vi "Select Data Items.vi"(10 "Page":i32, 11 "Data":T1(array[cluster])) -> (3 "subarray":string[][](array[string]))   [LabVIEW 2019, in "Full User Interface.lvlib"]
uses:
  Full User Interface.lvlib
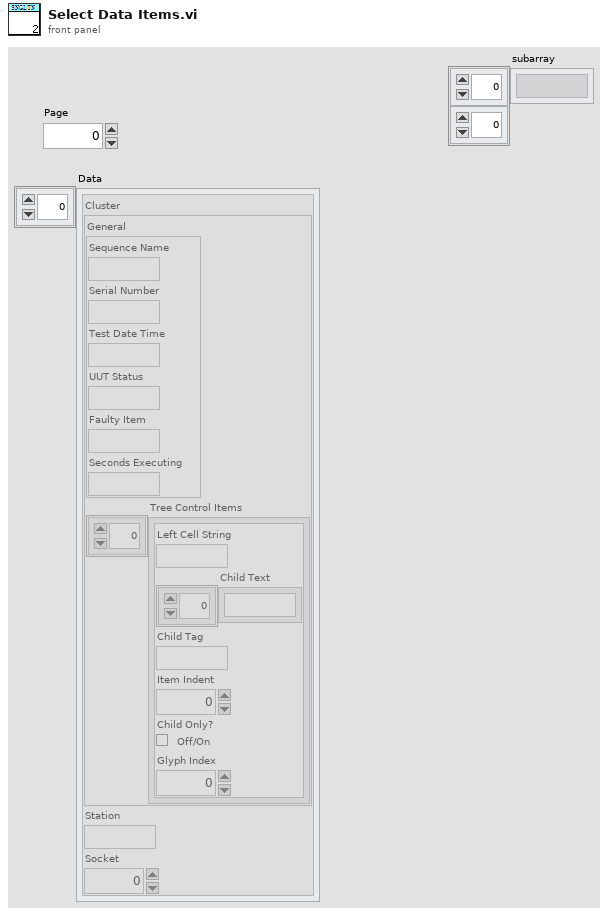
[diagram p1: front panel]
types:
  T1 = cluster{"Cluster":cluster{"General":cluster{"Sequence Name":string, "Serial Number":string, "Test Date Time":string, "UUT Status":string, "Faulty Item":string, "Seconds Executing":string}, "Tree Control Items":cluster{"Left Cell String":string, "Child Text":string[], "Child Tag":string, "Item Indent":i32, "Child Only?":bool, "Glyph Index":i32}[]}, "Station":string, "Socket":i32}[]
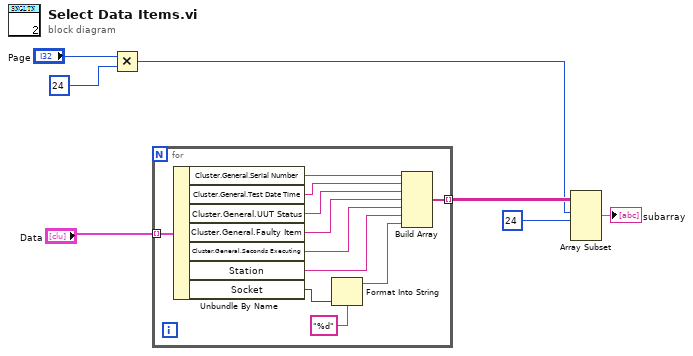
[diagram p0: block diagram]
diagram:
  n1 = Multiply(x="Page", y=24) -> (x*y=w2:i32)
  n2 = for {
    tunnel: "Data" -> [w18] mode=indexing
    tunnel: [w8] -> w6 mode=indexing
    n3 = Unbundle By Name(w18) -> ("Cluster.General.Serial Number"=w17:string, "Cluster.General.Test Date Time"=w16:string, "Cluster.General.UUT Status"=w15:string, "Cluster.General.Faulty Item"=w14:string, "Cluster.General.Seconds Executing"=w13:string, "Station"=w12:string, "Socket"=w11:i32)
    n4 = Format Into String(format string="%d", w11) -> (resulting string=w9:string)  [unwired: 2 in, 1 out]
    n5 = Build Array(w17, w16, w15, w14, w13, w12, w9) -> (w8:string[])
  }
  n6 = Array Subset(array=w6, index (row)=w2, length (row)=24 ("length")) -> (→"subarray":string[][])  [unwired: 2 in]
